vi "PDLM_GetPresetInfo.vi"(8 "error in (no error)":errorcluster, 10 "PsIdx":u32=1, 11 "USBIdx":i32) -> (0 "error out":errorcluster, 1 "PsInfo":string, 3 "return type":i32)   [LabVIEW 2017]
uses:
  PDLM_DllPath_global.vi
panel:
  in  "StrBuffer":string
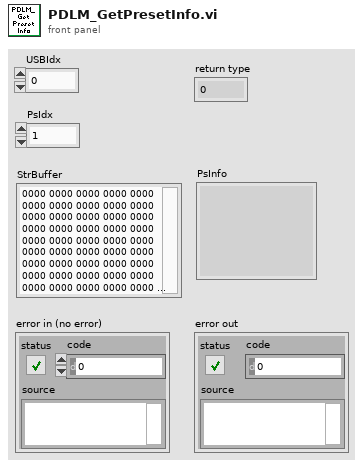
[diagram p1: front panel]
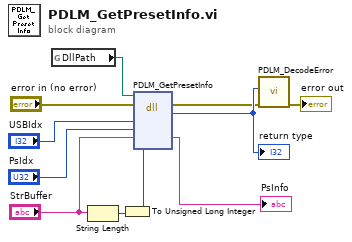
[diagram p0: block diagram]
diagram:
  n1 = global read "PDLM_DllPath_global.vi" "DllPath"() -> (w7:path)
  n2 = String Length(string="StrBuffer") -> (length=w4:i32)
  n3 = To Unsigned Long Integer(number=w4) -> (unsigned 32bit integer=w3:u32)
  n4 = dll-call lib="M:/_dev/progs/LabVIEW/_lib/PQ/Taiko/pdlm_lib.dll" fn="PDLM_GetPresetInfo"(path in=w7, error in="error in (no error)", "USBIdx"="USBIdx", "PsIdx"="PsIdx", "PsInfo"="StrBuffer", "size"=w3) -> (error out=w9:errorcluster, "return type"=w10:i32, "PsInfo"=→"PsInfo":string)  [unwired: 4 in, 1 out]
  "return type" <- w10
  n5 = call "PDLM_DecodeError.vi"("error in (no error)"=w9, "code"=w10) -> ("error out"=→"error out":errorcluster)  [unwired: 7 in, 2 out]
